vi "Set ESP Variable.vi"   [LabVIEW 2020, in "NI_WebServices.lvlib" / "Web Request.lvclass"]
doc: "Sets variables to be visible in an ESP scripting template. You can access these variables from the form variables in the ESP template. Refer to the Scripting in LabVIEW Web Services topic at ni.com for more information about using scripting with Web services. The data type you wire to the <B>value</B> input determines the polymorphic instance to use."
uses:
  <vilib>/wsapi/Web Request.lvclass
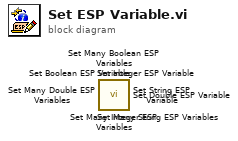
[diagram p0: block diagram]
diagram:
  n1 = call <vilib>:"Set Many Integer ESP Variables.vi"() -> ()  [unwired: 14 in, 2 out]
  n2 = call <vilib>:"Set Integer ESP Variable.vi"() -> ()  [unwired: 14 in, 2 out]
  n3 = call <vilib>:"Set Many Double ESP Variables.vi"() -> ()  [unwired: 14 in, 2 out]
  n4 = call <vilib>:"Set Double ESP Variable.vi"() -> ()  [unwired: 14 in, 2 out]
  n5 = call <vilib>:"Set Many Boolean ESP Variables.vi"() -> ()  [unwired: 14 in, 2 out]
  n6 = call <vilib>:"Set Boolean ESP Variable.vi"() -> ()  [unwired: 14 in, 2 out]
  n7 = call <vilib>:"Set Many String ESP Variables.vi"() -> ()  [unwired: 14 in, 2 out]
  n8 = call <vilib>:"Set String ESP Variable.vi"() -> ()  [unwired: 14 in, 2 out]
